vi "PH_Strings.Remove last zeros from a double number string.vi"(1 "String in":string) -> (0 "String out":string)   [LabVIEW 2014, in "PH_Common.lvlib"]
doc: "This VI acts on strings that are double numbers; it removes the last digits if these are zero."
uses:
  PH_Common.lvlib
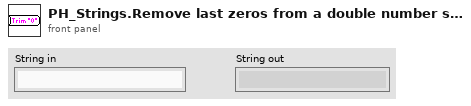
[diagram p1: front panel]
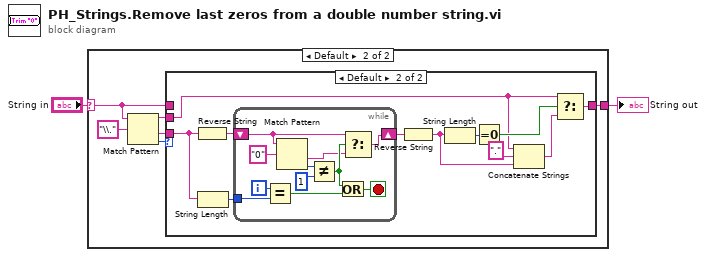
[diagram p0: block diagram]
diagram:
  n1 = case shown="Default" "String in" {
    selector: "String in" -> [w3 w5]
    tunnel: [w3 w9] -> w2
    frame "", "N/A" {
    }
    frame Default {
      n2 = Match Pattern(string=w5, regular expression="\\.") -> (before substring=w4:string, after substring=w7:string, offset past match=w6:i32)  [unwired: 1 in, 1 out]
      n3 = case shown="Default" w6 {
        tunnel: [w10 w12] -> w9
        tunnel: w5 -> [w10 _]
        tunnel: w7 -> [_ w18]
        tunnel: w4 -> [_ w11]
        frame -1 {
        }
        frame Default {
          n4 = Reverse String(1:w18) -> (0:w20:string)
          n5 = String Length(string=w18) -> (length=w19:i32)
          n6 = while {
            shift-right: [w27] -> w21
            shift-left: w20 -> [w26]
            tunnel: w19 -> [w23]
            i -> [w24]
            stop <- w30 stop-if-true
            n7 = Equal?(x=w24, y=w23) -> (x = y?=w25:bool)
            n8 = Match Pattern(string=w26, regular expression="0") -> (after substring=w28:string, offset past match=w32:i32)  [unwired: 1 in, 2 out]
            n9 = Not Equal?(x=w32, y=1) -> (x != y?=w29:bool)
            n10 = Or(x=w29, y=w25) -> (x .or. y?=w30:bool)
            n11 = Select(t=w26, s=w29, f=w28) -> (s? t:f=w27:string)
          }
          n12 = Reverse String(1:w21) -> (0:w16:string)
          n13 = String Length(string=w16) -> (length=w15:i32)
          n14 = Equal To 0?(x=w15) -> (x = 0?=w14:bool)
          n15 = Concatenate Strings(w11, "." ("string"), w16) -> (w13:string)
          n16 = Select(t=w11, s=w14, f=w13) -> (s? t:f=w12:string)
        }
      }
    }
  }
  "String out" <- w2
